vi "Write Receive Text Data.vi"(8 "error in (no error)":errorcluster, 9 "values":string, 10 "starting address":u16, 11 "standard data model in":refnum<class "WebSocket Data Model.lvclass">) -> (0 "error out":errorcluster, 3 "standard data model out":refnum<class "WebSocket Data Model.lvclass">)   [LabVIEW 2021, in "WebSockets.lvlib" / "WebSocket Data Model.lvclass"]
doc: "Writes the values of multiple input register values in series, starting at address M."
uses:
  WebSocket Data Model.lvclass
  WebSocket Data Model.lvclass/WebSocket Data Model.ctl
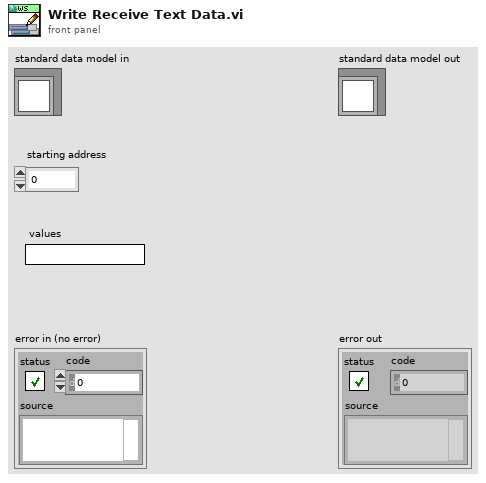
[diagram p1: front panel]
types:
  T1 = typedef "WebSockets.lvlib/WebSocket Data Model.lvclass/Data Model.ctl" = cluster{"UTC":u64, "Receive Binary Data":u8[], "Receive Text Data":string, "Send Binary Data":u8[], "Send Text Data":string, "ES":u8}
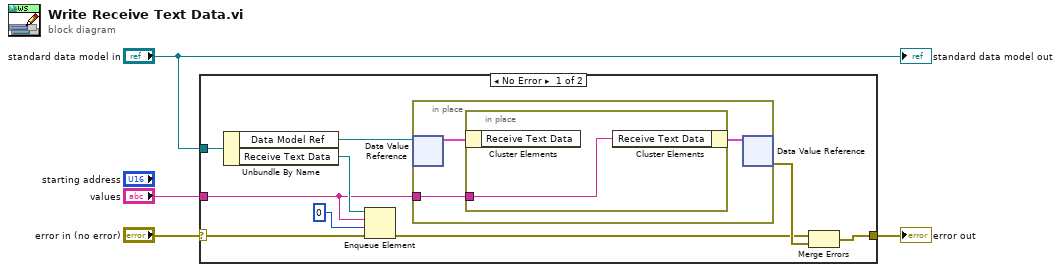
[diagram p0: block diagram]
diagram:
  n1 = case shown="No Error" "error in (no error)" {
    selector: "error in (no error)" -> [w7 w18]
    tunnel: "values" -> [w6 _]
    tunnel: "standard data model in" -> [w9 _]
    tunnel: [w13 w18] -> w2
    frame No Error {
      n2 = Unbundle By Name(w9) -> ("Data Model Ref"=w12:refnum<data-value>, "Receive Text Data"=w8:refnum<queue>)
      n3 = Enqueue Element(queue=w8, element=w6, timeout in ms (-1)=0, error in (no error)=w7) -> (error out=w5:errorcluster)  [unwired: 2 out]
      n4 = in-place {
        in-place-border: w6 -> [w16]
        n5 = in-place-dvr #1(w12) -> (w15:T1)  [unwired: 1 out]
        n6 = in-place {
          in-place-border: w16 -> [w17]
          n7 = in-place-cluster #2(w15) -> ()  [unwired: 1 out]
          n8 = in-place-cluster #2("Receive Text Data"=w17) -> (w14:T1)
        }
        n9 = in-place-dvr #1(w14) -> (w11:errorcluster)  [unwired: 1 out]
      }
      n10 = Merge Errors(w5, w11) -> (w13:errorcluster)
    }
    frame Error {
    }
  }
  "error out" <- w2
  "standard data model out" <- "standard data model in"
